vi "Odczyt temp wewn.vi"() -> ()   [LabVIEW 2014]
uses:
  <resource>/objmgr/daqmx.rc
panel:
  in  "stop":bool
  out "DevTemp":dbl
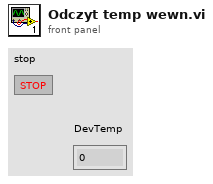
[diagram p1: front panel]
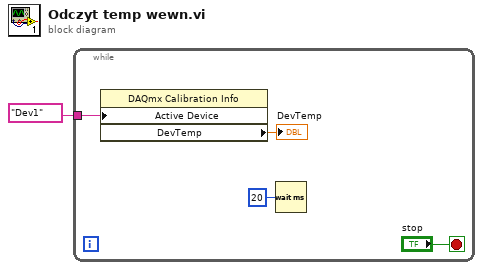
[diagram p0: block diagram]
diagram:
  n1 = while {
    tunnel: tag "Dev1" ("ActiveDev") -> [w5]
    stop <- "stop" stop-if-true
    n2 = property class="DAQmx Calibration Info"("Active Device"=w5) -> ("DevTemp"=→"DevTemp":dbl)  [unwired: 2 in, 2 out]
    n3 = Wait (ms)(milliseconds to wait=u32 20) -> ()  [unwired: 1 out]
  }
